vi "Add Port.vi"(4 "Baud Rate":u32, 6 "Database Path":path, 7 "Highlight? (F)":bool, 8 "error in":errorcluster, 9 "Database Name":string, 10 "Port Name":string, 11 "Ports Ref":T1 format="%.0x") -> (0 "error out":errorcluster, 3 "Port Ref out":T1 format="%.0x")   [LabVIEW 2020, in "Ballard ARINC 429 Scripting.lvlib"]
uses:
  Ballard ARINC 429 Scripting.lvlib
  <vilib>/NI VeriStand/Custom Device API/Custom Device API.lvlib
  Constants.vi
  <vilib>/NI VeriStand/Custom Device API/Custom Device Item Ref.ctl
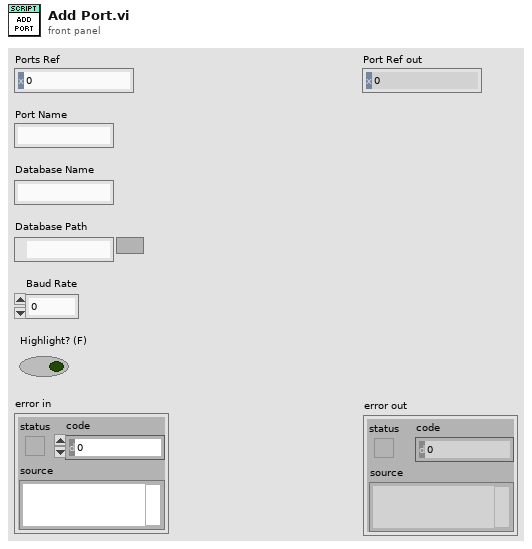
[diagram p1: front panel]
types:
  T1 = typedef "Custom Device API.lvlib/Custom Device Item Ref.ctl" = u64
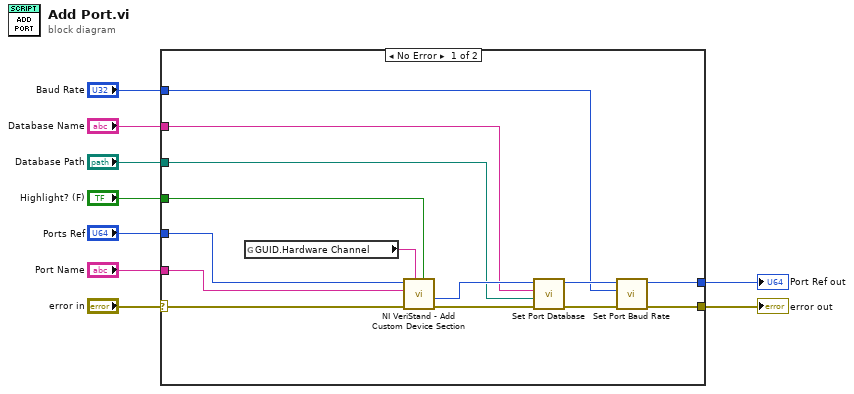
[diagram p0: block diagram]
diagram:
  n1 = case shown="No Error" "error in" {
    selector: "error in" -> [w19 w24]
    tunnel: "Highlight? (F)" -> [w22 _]
    tunnel: "Ports Ref" -> [w21 _]
    tunnel: [w11 w24] -> w7
    tunnel: "Database Name" -> [w16 _]
    tunnel: "Database Path" -> [w15 _]
    tunnel: "Baud Rate" -> [w10 _]
    tunnel: [w13 _] -> w3
    tunnel: "Port Name" -> [w20 _]
    frame No Error {
      n2 = global read "Constants.vi" "GUID.Hardware Channel"() -> (w23:string)
      n3 = call <vilib>:"NI VeriStand - Add Custom Device Section.vi"("Highlight? (F)"=w22, "GUID (Default Section)"=w23, "error in (no error)"=w19, "Section Name"=w20, "Parent Ref in"=w21) -> ("error out"=w17:errorcluster, "Section Ptr"=w18:T1)  [unwired: 3 in, 2 out]
      n4 = call "Set Port Database.vi"("error in"=w17, "Database Path"=w15, "Database Name"=w16, "Port Ref"=w18) -> ("error out"=w12:errorcluster, "Port Ref out"=w14:T1)  [unwired: 6 in]
      n5 = call "Set Port Baud Rate.vi"("error in"=w12, "Baud Rate"=w10, "Port Ref"=w14) -> ("error out"=w11:errorcluster, "Port Ref out"=w13:T1)  [unwired: 7 in]
    }
    frame Error {
    }
  }
  "error out" <- w7
  "Port Ref out" <- w3
